vi "osciJSON.vi"(8 "Error in (no error)":errorcluster, 11 "Application ref in":refnum<vi>) -> (0 "Error out":errorcluster, 2 "JSON string":string, 3 "Application ref out":refnum<vi>)   [LabVIEW 2021]
uses:
  <userlib>/Nanonis Prog Interface V5/Nanonis Prog Interface.lvlib
panel:
  out "Range":enum16{"10", "1", "0.1", "0.01", "0.001"}(ring)=enum."1" caption="Output range (V)"
  in  "PLL":T1={"Excitation (V)"=0.0, "Differential input"=FALSE, "1/10 Divider"=FALSE, "Input range (m)"=0.0, "Calibration (m/V)"=0.0, "Amplitude Controller Time constant (s)"=0.0, "Amplitude Controller P-gain"=0.0, "Amplitude Controller I-gain"=0.0, "Amplitude Controller Bandwidth (Hz)"=0.0, "Frequency range (Hz)"=0.0, "Center Frequency (Hz)"=0.0, "Phase Controller P-gain"=0.0, "Phase Controller Time constant (s)"=0.0, "Phase Controller I-gain"=0.0, "Phase Controller Bandwidth (Hz)"=0.0, "Phase reference (deg)"=0.0, "Cutoff Frq (Hz)"=0.0, "Filter Order (1...8)"=1, "Harmonic (1, ...) out"=1, "Range"="", "Amplitude (m)"=0.0} {"Amplitude (m)" format="%#_6p"; "Harmonic (1, ...) out" min=1 max=16 step=1; "Filter Order (1...8)" min=1 max=16 step=1; "Phase reference (deg)" format="%#_6p"; "Center Frequency (Hz)" format="%#_6p"; "Frequency range (Hz)" format="%#_6p"; "Calibration (m/V)" format="%#_6p"; "Input range (m)" min=0 format="%#_6p"; "Excitation (V)" format="%#_6p"}
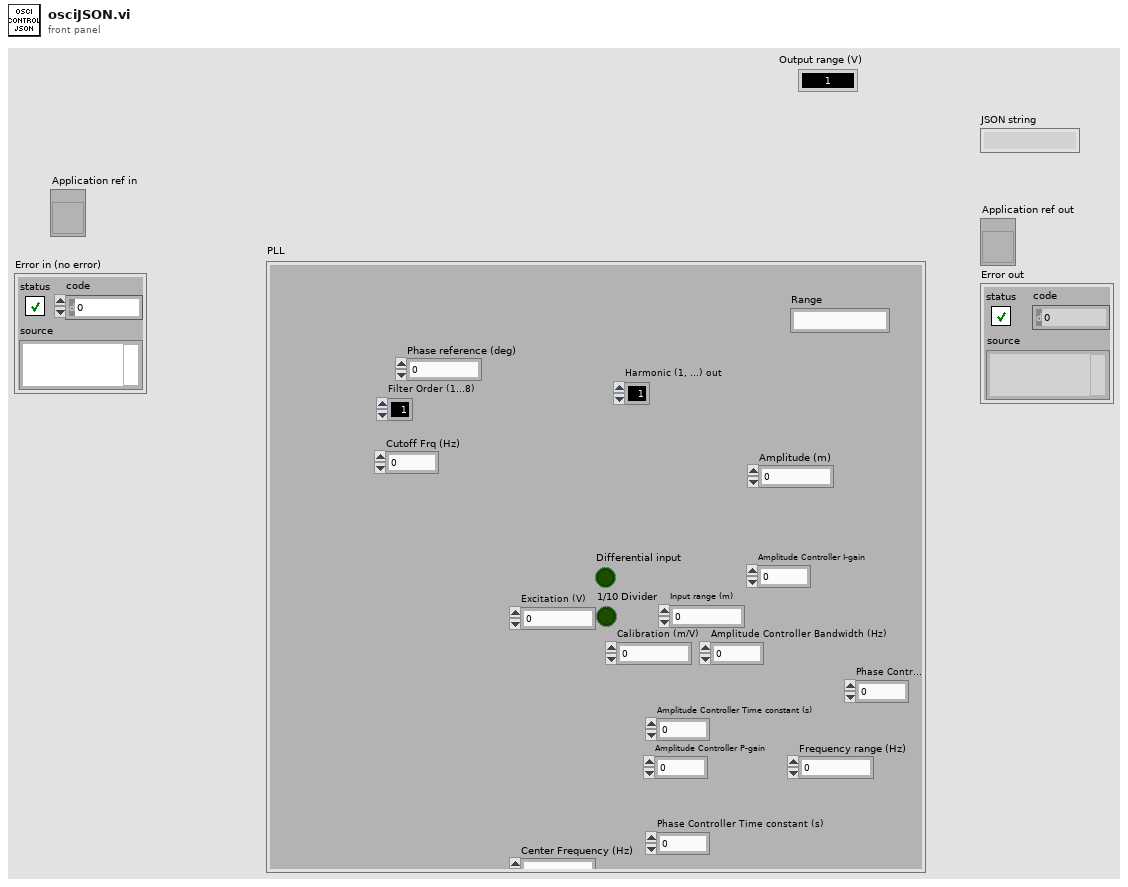
[diagram p1: front panel]
types:
  T1 = cluster{"Excitation (V)":sgl, "Differential input":bool, "1/10 Divider":bool, "Input range (m)":sgl, "Calibration (m/V)":sgl, "Amplitude Controller Time constant (s)":sgl, "Amplitude Controller P-gain":sgl, "Amplitude Controller I-gain":sgl, "Amplitude Controller Bandwidth (Hz)":sgl, "Frequency range (Hz)":sgl, "Center Frequency (Hz)":dbl, "Phase Controller P-gain":sgl, "Phase Controller Time constant (s)":sgl, "Phase Controller I-gain":sgl, "Phase Controller Bandwidth (Hz)":sgl, "Phase reference (deg)":sgl, "Cutoff Frq (Hz)":sgl, "Filter Order (1...8)":u16, "Harmonic (1, ...) out":u32, "Range":string, "Amplitude (m)":sgl}
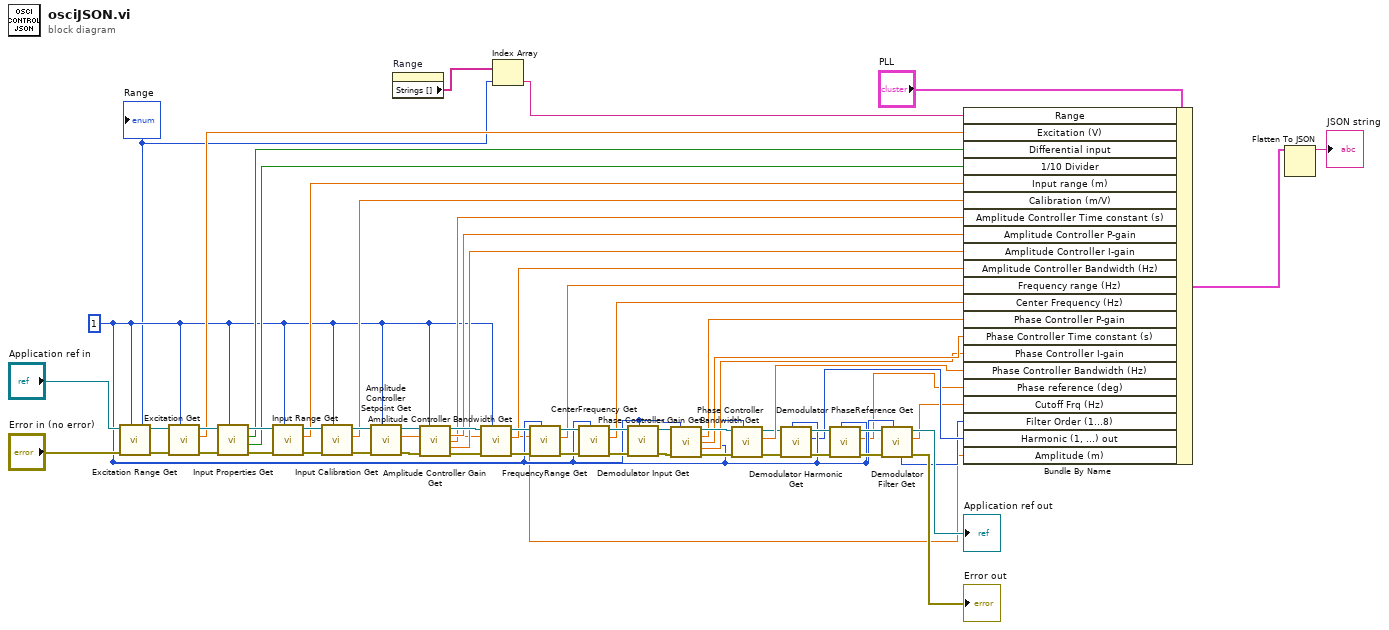
[diagram p0: block diagram]
diagram:
  w12 = 1 ("Modulator index")
  n1 = call <userlib>:"Excitation Range Get.vi"("Modulator index"=w12, "Error in (no error)"="Error in (no error)", "Application ref in"="Application ref in") -> ("Error out"=w58:errorcluster, "Range"=w3:enum16{"10", "1", "0.1", "0.01", "0.001"}, "Application ref out"=w57:refnum<vi>)  [unwired: 6 in]
  "Range" <- w3
  n2 = call <userlib>:"Excitation Get.vi"("Modulator index"=w12, "Error in (no error)"=w58, "Application ref in"=w57) -> ("Error out"=w56:errorcluster, "Excitation (V)"=w33:sgl, "Application ref out"=w55:refnum<vi>)  [unwired: 6 in]
  n3 = call <userlib>:"Input Properties Get.vi"("Modulator index"=w12, "Error in (no error)"=w56, "Application ref in"=w55) -> ("Error out"=w54:errorcluster, "1/10 Divider"=w31:bool, "Differential input"=w32:bool, "Application ref out"=w53:refnum<vi>)  [unwired: 5 in]
  n4 = call <userlib>:"Input Range Get.vi"("Modulator index"=w12, "Error in (no error)"=w54, "Application ref in"=w53) -> ("Error out"=w52:errorcluster, "Input range (m)"=w30:sgl, "Application ref out"=w51:refnum<vi>)  [unwired: 6 in]
  n5 = call <userlib>:"Input Calibration Get.vi"("Modulator index"=w12, "Error in (no error)"=w52, "Application ref in"=w51) -> ("Error out"=w50:errorcluster, "Calibration (m/V)"=w29:sgl, "Application ref out"=w49:refnum<vi>)  [unwired: 6 in]
  n6 = call <userlib>:"Amplitude Controller Setpoint Get.vi"("Modulator index"=w12, "Error in (no error)"=w50, "Application ref in"=w49) -> ("Error out"=w47:errorcluster, "Amplitude (m)"=w1:sgl, "Application ref out"=w48:refnum<vi>)  [unwired: 6 in]
  n7 = property on="Range" class="Enum (strict)"() -> ("Strings []"=w4:string[])  [unwired: 2 in, 2 out]
  n8 = call <userlib>:"Amplitude Controller Gain Get.vi"("Application ref in"=w48, "Modulator index"=w12, "Error in (no error)"=w47) -> ("Application ref out"=w45:refnum<vi>, "P-gain"=w28:sgl, "Time constant (s)"=w27:sgl, "I-gain"=w26:sgl, "Error out"=w46:errorcluster)  [unwired: 8 in]
  n9 = call <userlib>:"Amplitude Controller Bandwidth Get.vi"("Modulator index"=w12, "Error in (no error)"=w46, "Application ref in"=w45) -> ("Error out"=w44:errorcluster, "Amplitude Controller Bandwidth (Hz)"=w25:sgl, "Application ref out"=w43:refnum<vi>)  [unwired: 6 in]
  n10 = Index Array(array=w4, index=w3) -> (element=w2:string)
  n11 = call <userlib>:"FrequencyRange Get.vi"("Modulator index"=w12, "Error in (no error)"=w44, "Application ref in"=w43) -> ("Error out"=w42:errorcluster, "Frequency range (Hz)"=w24:sgl, "Application ref out"=w41:refnum<vi>)  [unwired: 6 in]
  n12 = call <userlib>:"CenterFrequency Get.vi"("Modulator index"=w12, "Error in (no error)"=w42, "Application ref in"=w41) -> ("Error out"=w40:errorcluster, "Center Frequency (Hz)"=w23:dbl, "Application ref out"=w39:refnum<vi>)  [unwired: 6 in]
  n13 = call <userlib>:"Demodulator Input Get.vi"("Demodulator index"=w12, "Error in (no error)"=w40, "Application ref in"=w39) -> ("Error out"=w37:errorcluster, "Application ref out"=w38:refnum<vi>)  [unwired: 5 in, 2 out]
  n14 = call <userlib>:"Phase Controller Gain Get.vi"("Application ref in"=w38, "Modulator index"=w12, "Error in (no error)"=w37) -> ("Application ref out"=w35:refnum<vi>, "P-gain"=w22:sgl, "Time constant (s)"=w21:sgl, "I-gain"=w20:sgl, "Error out"=w36:errorcluster)  [unwired: 8 in]
  n15 = call <userlib>:"Phase Controller Bandwidth Get.vi"("Modulator index"=w12, "Error in (no error)"=w36, "Application ref in"=w35) -> ("Error out"=w18:errorcluster, "Phase Controller Bandwidth (Hz)"=w19:sgl, "Application ref out"=w17:refnum<vi>)  [unwired: 6 in]
  n16 = call <userlib>:"Demodulator Harmonic Get.vi"("Demodulator index"=w12, "Error in (no error)"=w18, "Application ref in"=w17) -> ("Error out"=w16:errorcluster, "Harmonic (1, ...) out"=w9:u32, "Application ref out"=w15:refnum<vi>)  [unwired: 6 in]
  n17 = call <userlib>:"Demodulator PhaseReference Get.vi"("Demodulator index"=w12, "Error in (no error)"=w16, "Application ref in"=w15) -> ("Error out"=w14:errorcluster, "Phase reference (deg)"=w8:sgl, "Application ref out"=w13:refnum<vi>)  [unwired: 6 in]
  n18 = call <userlib>:"Demodulator Filter Get.vi"("Demodulator index"=w12, "Error in"=w14, "Application ref in"=w13) -> ("Error out"=→"Error out":errorcluster, "Cutoff Frq (Hz)"=w7:sgl, "Application ref out"=→"Application ref out":refnum<vi>, "Filter Order (1...8)"=w6:u16)  [unwired: 4 in, 1 out]
  n19 = Bundle By Name(cluster="PLL", "Range"=w2, "Excitation (V)"=w33, "Differential input"=w32, "1/10 Divider"=w31, "Input range (m)"=w30, "Calibration (m/V)"=w29, "Amplitude Controller Time constant (s)"=w27, "Amplitude Controller P-gain"=w28, "Amplitude Controller I-gain"=w26, "Amplitude Controller Bandwidth (Hz)"=w25, "Frequency range (Hz)"=w24, "Center Frequency (Hz)"=w23, "Phase Controller P-gain"=w22, "Phase Controller Time constant (s)"=w21, "Phase Controller I-gain"=w20, "Phase Controller Bandwidth (Hz)"=w19, "Phase reference (deg)"=w8, "Cutoff Frq (Hz)"=w7, "Filter Order (1...8)"=w6, "Harmonic (1, ...) out"=w9, "Amplitude (m)"=w1) -> (w5:T1)
  n20 = Flatten To JSON(anything=w5) -> (JSON string=→"JSON string":string)  [unwired: 2 in, 1 out]
